vi "DriveForward.vi"(8 "Backward?":bool, 9 "Distance":dbl, 11 "Boolean in":bool) -> (3 "Boolean out":bool)   [LabVIEW 2014]
uses:
  Support Files/Global Data!!!.vi
  <vilib>/addons/control/pid/pid.llb/PID (DBL).vi
  <vilib>/addons/control/pid/NI_PID_pid.lvlib
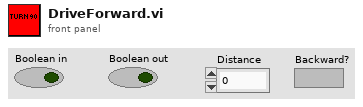
[diagram p1: front panel]
types:
  T1 = cluster{"proportional gain (Kc)":dbl, "integral time (Ti, min)":dbl, "derivative time (Td, min)":dbl}
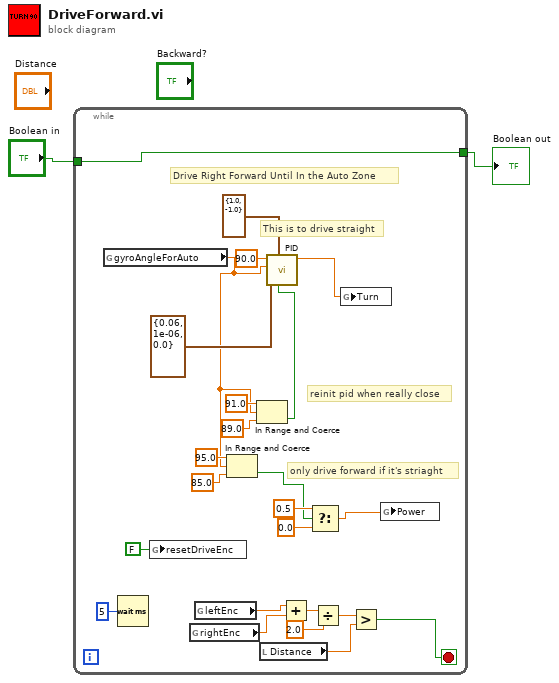
[diagram p0: block diagram]
diagram:
  n1 = while {
    tunnel: [w4] -> w1
    tunnel: "Boolean in" -> [w4]
    stop <- w9 stop-if-true
    # "reinit pid when really close"
    # "Drive Right Forward Until In the Auto Zone"
    # "only drive forward if it's striaght"
    # "This is to drive straight"
    n2 = global read "Global Data!!!.vi" "gyroAngleForAuto"() -> (w6:dbl)
    n3 = Wait (ms)(milliseconds to wait=u32 5) -> ()  [unwired: 1 out]
    n4 = global write "Global Data!!!.vi" "resetDriveEnc"(FALSE ("resetDriveEnc")) -> ()
    n5 = global read "Global Data!!!.vi" "rightEnc"() -> (w13:dbl)
    n6 = global read "Global Data!!!.vi" "leftEnc"() -> (w14:dbl)
    n7 = In Range and Coerce(upper limit=95.0, x=w6, lower limit=85.0) -> (In Range?=w16:bool)  [unwired: 1 out]
    n8 = In Range and Coerce(upper limit=91.0, x=w6, lower limit=89.0) -> (In Range?=w5:bool)  [unwired: 1 out]
    n9 = local read "Distance"() -> (w3:dbl)
    n10 = call-poly <vilib>:"PID.vi"("reinitialize? (F)"=w5, "output range"=cluster{"output high":dbl, "output low":dbl} {"output high"=1.0, "output low"=-1.0}, "PID gains"=T1 {"proportional gain (Kc)"=0.06, "integral time (Ti, min)"=1e-06, "derivative time (Td, min)"=0.0}, "process variable"=w6, "setpoint"=90.0) -> ("output"=w24:dbl)  [unwired: 5 in, 1 out]
    n11 = Add(x=w14, y=w13) -> (x+y=w12:dbl)
    n12 = Select(t=0.5, s=w16, f=0.0) -> (s? t:f=w21:dbl)
    n13 = Divide(x=w12, y=2.0) -> (x/y=w10:dbl)
    n14 = global write "Global Data!!!.vi" "Turn"(w24) -> ()
    n15 = Greater?(x=w10, y=w3) -> (0:w9:bool)
    n16 = global write "Global Data!!!.vi" "Power"(w21) -> ()
  }
  "Boolean out" <- w1
